vi "U8_3_byte_Array_to_voltage_current.vi"(5 "CH0 Shift V":dbl, 7 "CH1 Shift V":dbl, 8 "CH0 multiplier":dbl, 9 "CH1 multiplier":dbl, 10 "Array In":u8[](array[numeric]), 11 "Nmbr_of_datasamples":dbl=128.0) -> (0 "Current":dbl[](graph), 1 "mV":dbl, 2 "Voltage":dbl[](graph), 3 "Loop count":dbl, 4 "COM":dbl[](graph), 6 "HEXVAL":string)   [LabVIEW 2012]
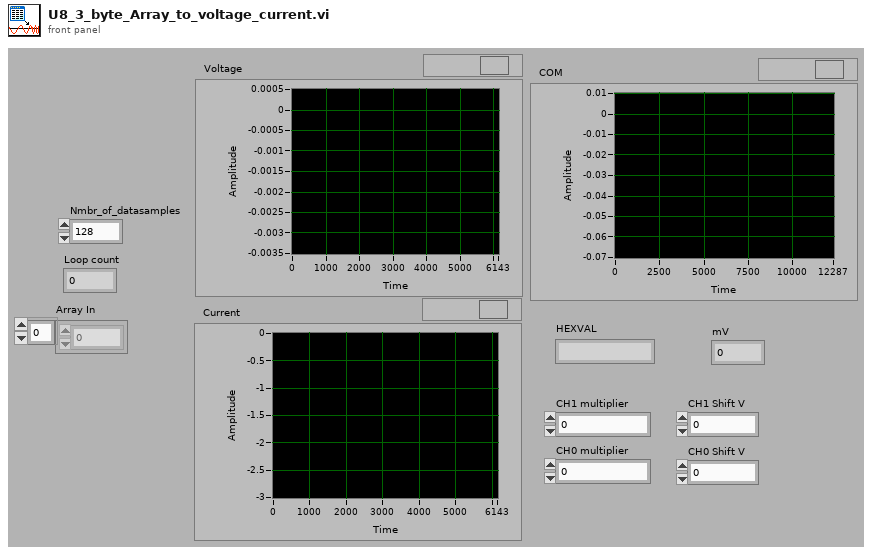
[diagram p1: front panel]
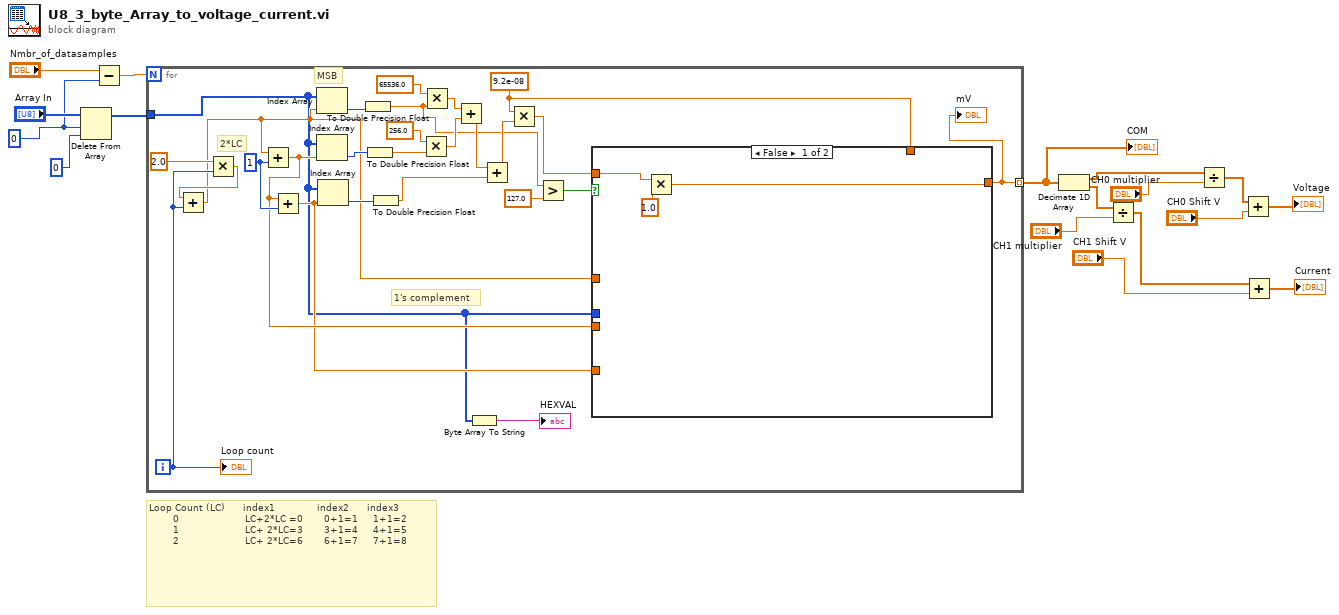
[diagram p0: block diagram]
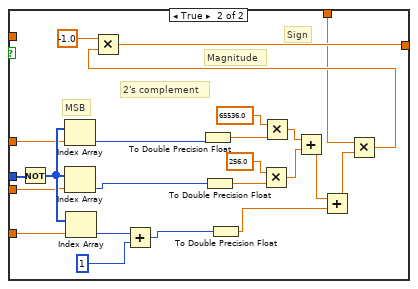
[diagram p2: hidden frame]
diagram:
  w13 = 0
  # "Loop Count (LC)      index1              index2      index3      \n        0                      LC+2*LC =0       0+1=1     1+1=2\n        1                      LC+ 2*LC=3       3+1=4     4+1=5\n        2                      LC+ 2*LC=6       6+1=7     7+1=8"
  n1 = Delete From Array(array="Array In", length=w13, index=0) -> (array with subset deleted=w12:u8[])  [unwired: 1 out]
  n2 = Subtract(x="Nmbr_of_datasamples", y=w13) -> (x-y=w15:dbl)
  n3 = for {
    N: w15 -> [_]
    tunnel: w12 -> [w18]
    tunnel: [w20] -> w11 mode=indexing
    i -> [w25]
    w24 = 9.2e-08
    w35 = 1
    # "1's complement"
    # "MSB"
    # "2*LC"
    n4 = Multiply(x=2.0, y=w25) -> (x*y=w33:dbl)
    n5 = Add(x=w33, y=w25) -> (x+y=w23:dbl)
    n6 = Add(x=w23, y=w35) -> (x+y=w22:dbl)
    n7 = Add(x=w22, y=w35) -> (x+y=w21:dbl)
    n8 = Index Array(array=w18, index=w23) -> (element=w28:u8)
    n9 = Index Array(array=w18, index=w22) -> (element=w27:u8)
    n10 = Index Array(array=w18, index=w21) -> (element=w26:u8)
    n11 = To Double Precision Float(number=w28) -> (double precision float=w29:dbl)
    n12 = To Double Precision Float(number=w27) -> (double precision float=w41:dbl)
    n13 = To Double Precision Float(number=w26) -> (double precision float=w37:dbl)
    n14 = Multiply(x=256.0, y=w41) -> (x*y=w39:dbl)
    n15 = Multiply(x=65536.0, y=w29) -> (x*y=w43:dbl)
    n16 = Add(x=w43, y=w39) -> (x+y=w38:dbl)
    n17 = Byte Array To String(unsigned byte array=w18) -> (string=→"HEXVAL":string)
    n18 = Add(x=w38, y=w37) -> (x+y=w36:dbl)
    n19 = Multiply(x=w24, y=w36) -> (x*y=w32:dbl)
    n20 = Greater?(x=w29, y=127.0) -> (0:w31:bool)
    n21 = case shown="False" w31 {
      tunnel: [w46 w69] -> w20
      tunnel: w32 -> [w45 _]
      tunnel: w18 -> [_ w56]
      tunnel: w23 -> [_ w51]
      tunnel: w22 -> [_ w50]
      tunnel: w21 -> [_ w49]
      tunnel: w24 -> [_ w47]
      frame False {
        n22 = Multiply(x=w45, y=1.0) -> (x*y=w46:dbl)
      }
      frame True {
        # "Magnitude"
        # "Sign"
        # "2's complement"
        # "MSB"
        n23 = Not(x=w56) -> (.not. x?=w55:u8[])
        n24 = Index Array(array=w55, index=w51) -> (element=w58:u8)
        n25 = Index Array(array=w55, index=w50) -> (element=w57:u8)
        n26 = Index Array(array=w55, index=w49) -> (element=w54:u8)
        n27 = Add(x=w54, y=1) -> (x+y=w52:i32)
        n28 = To Double Precision Float(number=w58) -> (double precision float=w59:dbl)
        n29 = To Double Precision Float(number=w57) -> (double precision float=w65:dbl)
        n30 = To Double Precision Float(number=w52) -> (double precision float=w61:dbl)
        n31 = Multiply(x=256.0, y=w65) -> (x*y=w63:dbl)
        n32 = Multiply(x=65536.0, y=w59) -> (x*y=w67:dbl)
        n33 = Add(x=w67, y=w63) -> (x+y=w62:dbl)
        n34 = Add(x=w62, y=w61) -> (x+y=w60:dbl)
        n35 = Multiply(x=w47, y=w60) -> (x*y=w48:dbl)
        n36 = Multiply(x=-1.0, y=w48) -> (x*y=w69:dbl)
      }
    }
    "mV" <- w20
    "Loop count" <- w25
  }
  "COM" <- w11
  n37 = Decimate 1D Array(w11) -> (w8:dbl[], w10:dbl[])
  n38 = Divide(x=w10, y="CH1 multiplier") -> (x/y=w1:dbl[])
  n39 = Divide(x=w8, y="CH0 multiplier") -> (x/y=w7:dbl[])
  n40 = Add(x=w7, y="CH0 Shift V") -> (x+y=→"Voltage":dbl[])
  n41 = Add(x=w1, y="CH1 Shift V") -> (x+y=→"Current":dbl[])
